vi "TimmingGraph.vi"(9 "lock":dbl, 10 "Cluster":T1) -> (0 "Waveform Graph 4":dynamicdata(graph), 1 "Waveform Graph 3":dynamicdata(graph), 2 "Waveform Graph 2":dynamicdata(graph), 3 "Waveform Graph":dynamicdata(graph))   [LabVIEW 2011]
uses:
  <vilib>/imath/engines/lvmath2/RunTimeEngine/ErrorHandling/NIMS_Finalize Error.vi
  <vilib>/imath/engines/lvmath2/RunTimeEngine/Managers/WorkSpace/UID Generator.vi
  <vilib>/imath/engines/lvmath2/RunTimeEngine/Managers/SymbolTable/Clear UID.vi
  <vilib>/imath/engines/lvmath2/RunTimeEngine/NodeEndStatement/NIMS_NodeEndStatement_Output.vi
  <instcachedir>/0/NIMS_NodeEndStatement_Output_53EC0D466D134D7ABD903AC30B43404B.lvgen/NIMS_NodeEndStatement_Output_53EC0D466D134D7ABD903AC30B43404B_002.vi
  <vilib>/imath/engines/lvmath2/RunTimeEngine/RunTimeType/NIMS_RunTimeType_From StrictType (excl LVString).vi
  <instcachedir>/0/NIMS_RunTimeType_From StrictType (excl LVString)_324186E61FB03FEA40CF23447A88CB3F.lvgen/NIMS_RunTimeType_From StrictType (excl LVString)_324186E61FB03FEA40CF23447A88CB3F_000.vi
  <vilib>/imath/engines/lvmath2/RunTimeEngine/LocalVariableDefStatement/MC_LocalVariableDefStatement_Display.vi
  <vilib>/imath/engines/lvmath2/RunTimeEngine/Managers/SymbolTable/NIMS_WorkSpace.lvlib
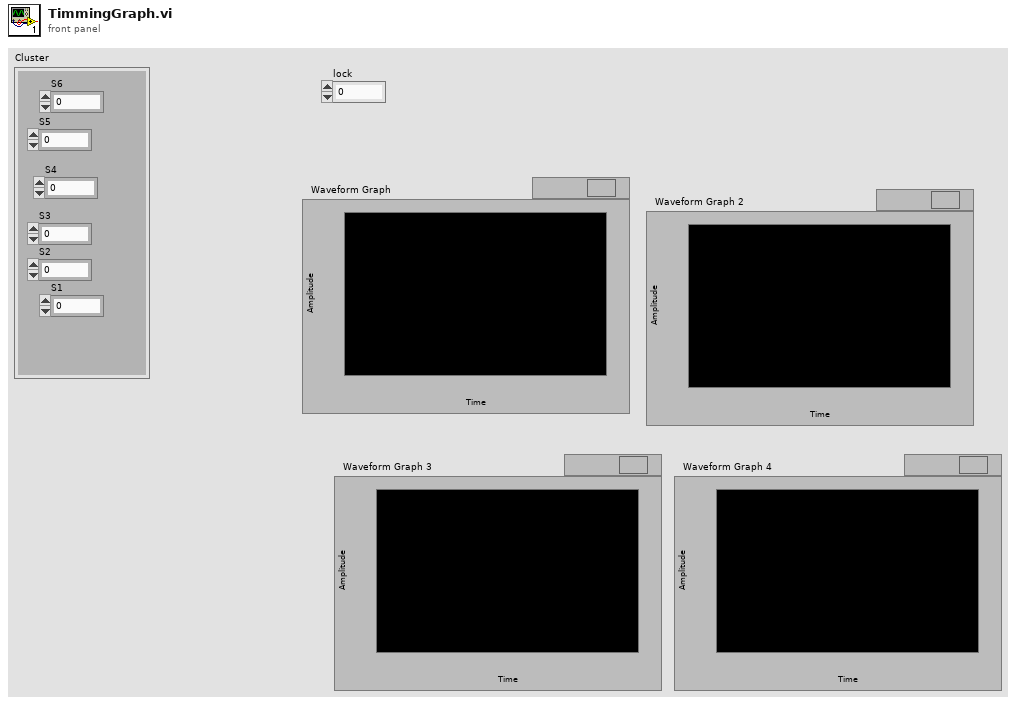
[diagram p1: front panel]
types:
  T1 = cluster{"S6":dbl, "S5":dbl, "S4":dbl, "S3":dbl, "S2":dbl, "S1":dbl}
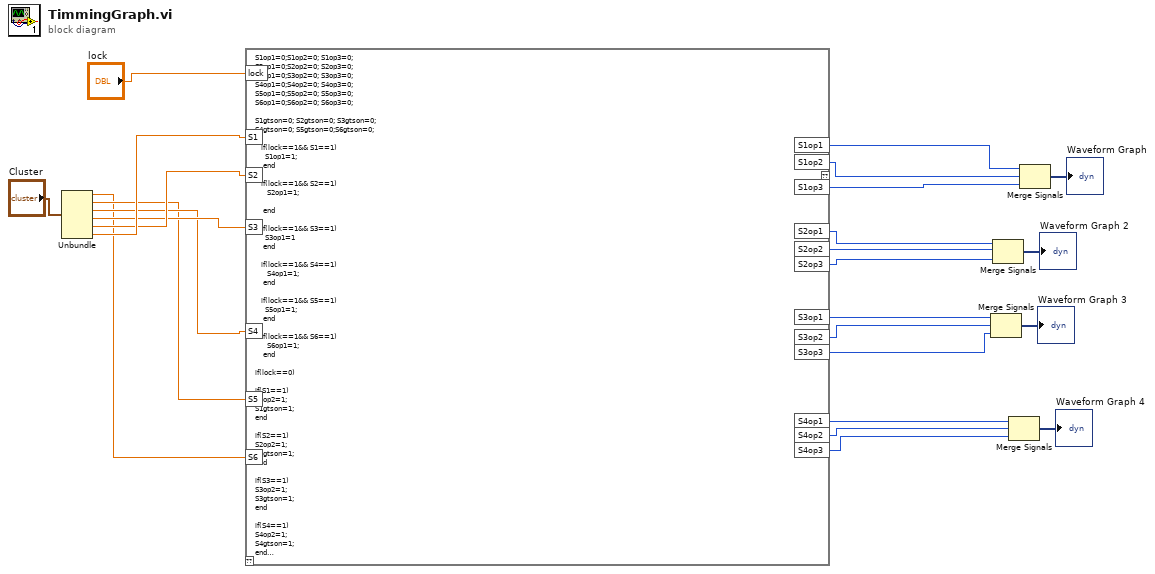
[diagram p0: block diagram]
diagram:
  n1 = Unbundle("Cluster") -> ("S6"=w13:dbl, "S5"=w14:dbl, "S4"=w15:dbl, "S3"=w16:dbl, "S2"=w17:dbl, "S1"=w18:dbl)
  n2 = mathscript code="S1op1=0;S1op2=0; S1op3=0;\nS2op1=0;S2op2=0; S2op3=0;\nS3op1=0;S3op2=0; S3op3=0;\nS4op1=0;S4op2=0; S4op3=0;\nS5op1=0;S5op2=0; S5op3=0;\nS6op1=0;S6op2=0; S6op3=0;\n\nS1gtson=0; S2gtson=0; S3gtson=0;\nS4gtson=0; S5gtson=0;S6gtson=0;\n\n   if(lock==1&& S1==1)\n     S1op1=1; \n    end\n\n   if(lock==1&& S2==1)\n      S2op1=1; \n     \n    end\n\n   if(lock==1&& S3==1)\n     S3op1=1\n    end\n\n   if(lock==1&& S4==1)\n      S4op1=1; \n    end\n\n   if(lock==1&& S5==1)\n     S5op1=1; \n    end\n\n   if(lock==1&& S6==1)\n      S6op1=1;\n    end    \n\nif(lock==0)\n\nif(S1==1)\nS1op2=1;\nS1gtson=1;\nend\n\nif(S2==1)\nS2op2=1;\nS2gtson=1;\nend\n\nif(S3==1)\nS3op2=1;\nS3gtson=1;\nend\n\nif(S4==1)\nS4op2=1;\nS4gtson=1;\nend\n\nif(S5==1)\nS5op2=1;\nS5gtson=1;\nend\n\nif(S6==1)\nS6op2=1;\nS6gtson=1;\nend\n \nend\n\n    \n\n\nif(S1==1&&S1gtson==1)\n   S1op3=1;\nend\n\nif(S2==1&&S2gtson==1)\n   S2op3=1;\nend\nif(S3==1&&S3gtson==1)\n   S3op3=1;\nend\nif(S4==1&&S4gtson==1)\n   S4op3=1;\nend\nif(S5==1&&S5gtson==1)\n   S5op3=1;\nend\nif(S6==1&&S6gtson==1)\n   S6op3=1;\nend"("lock"="lock", "S1"=w18, "S2"=w17, "S3"=w16, "S4"=w15, "S5"=w14, "S6"=w13) -> ("S1op1"=w24:i32, "S1op2"=w23:i32, "S1op3"=w22:i32, "S2op1"=w9:i32, "S2op2"=w8:i32, "S2op3"=w7:i32, "S3op1"=w6:i32, "S3op2"=w5:i32, "S3op3"=w4:i32, "S4op1"=w3:i32, "S4op2"=w2:i32, "S4op3"=w1:i32)  [unwired: 1 in, 1 out]
  n3 = Merge Signals(w6, w5, w4) -> (→"Waveform Graph 3":dynamicdata)
  n4 = Merge Signals(w9, w8, w7) -> (→"Waveform Graph 2":dynamicdata)
  n5 = Merge Signals(w3, w2, w1) -> (→"Waveform Graph 4":dynamicdata)
  n6 = Merge Signals(w24, w23, w22) -> (→"Waveform Graph":dynamicdata)
